vi "SetLimitTripOffLCDC501.vi"(2 "LASER LIMIT & TRIP-OFF":T1, 8 "error in (no error)":errorcluster, 11 "VISA resource name":refnum<visa-resource-name>) -> (0 "error out":errorcluster, 3 "VISA resource name out":refnum<visa-resource-name>)   [LabVIEW 2021]
panel:
  # "Laser Trip-off on"
  # "Current Limit"
  # "TEC Off"
  # "Min Temperature"
  # "Max Temperature"
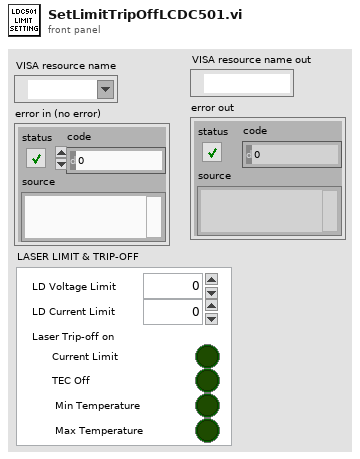
[diagram p1: front panel]
types:
  T1 = cluster{"LD Voltage Limit":dbl, "LD Current Limit":dbl, "Laser Trip-off on Current Limit":bool, "Laser Trip-off on TEC Off":bool, "Laser Trip-off on Min Temperature":bool, "Laser Trip-off on Max Temperature":bool}
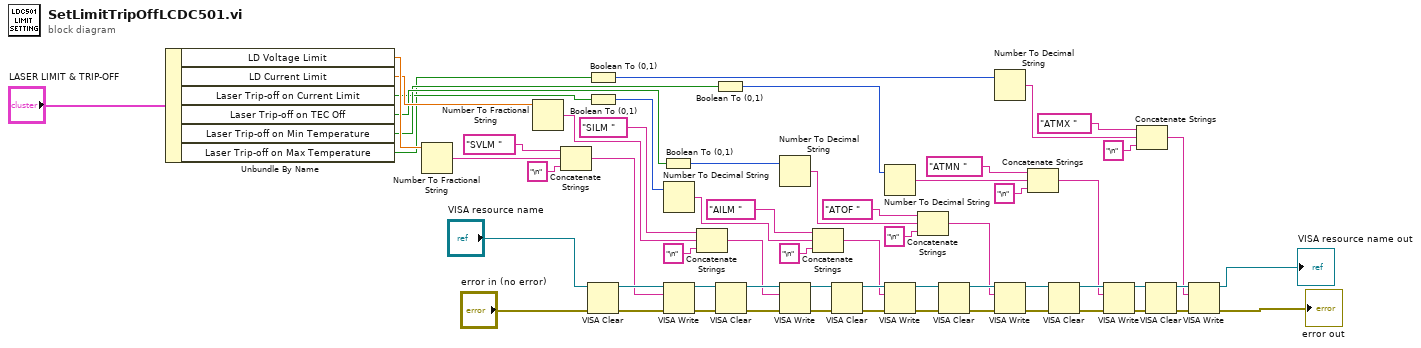
[diagram p0: block diagram]
diagram:
  n1 = Unbundle By Name("LASER LIMIT & TRIP-OFF") -> ("LD Voltage Limit"=w46:dbl, "LD Current Limit"=w45:dbl, "Laser Trip-off on Current Limit"=w42:bool, "Laser Trip-off on TEC Off"=w44:bool, "Laser Trip-off on Min Temperature"=w43:bool, "Laser Trip-off on Max Temperature"=w41:bool)
  n2 = Number To Fractional String(number=w46) -> (F-format string=w36:string)  [unwired: 3 in]
  n3 = Number To Fractional String(number=w45) -> (F-format string=w31:string)  [unwired: 3 in]
  n4 = Concatenate Strings("SVLM " ("write buffer"), w36, "\n" ("string")) -> (w33:string)
  n5 = Boolean To (0,1)(Boolean=w41) -> (0, 1=w37:i16)
  n6 = Boolean To (0,1)(Boolean=w42) -> (0, 1=w40:i16)
  n7 = VISA Clear(VISA resource name="VISA resource name", error in (no error)="error in (no error)") -> (VISA resource name out=w60:refnum<visa-resource-name>, error out=w61:errorcluster)
  n8 = Boolean To (0,1)(Boolean=w44) -> (0, 1=w39:i16)
  n9 = Number To Decimal String(number=w40) -> (decimal integer string=w22:string)  [unwired: 1 in]
  n10 = VISA Write(VISA resource name=w60, write buffer=w33, error in (no error)=w61) -> (VISA resource name out=w29:refnum<visa-resource-name>, error out=w28:errorcluster)  [unwired: 1 out]
  n11 = Concatenate Strings("SILM " ("write buffer"), w31, "\n" ("string")) -> (w27:string)
  n12 = Boolean To (0,1)(Boolean=w43) -> (0, 1=w38:i16)
  n13 = VISA Clear(VISA resource name=w29, error in (no error)=w28) -> (VISA resource name out=w58:refnum<visa-resource-name>, error out=w59:errorcluster)
  n14 = Number To Decimal String(number=w39) -> (decimal integer string=w17:string)  [unwired: 1 in]
  n15 = VISA Write(VISA resource name=w58, write buffer=w27, error in (no error)=w59) -> (VISA resource name out=w26:refnum<visa-resource-name>, error out=w25:errorcluster)  [unwired: 1 out]
  n16 = Concatenate Strings("AILM " ("write buffer"), w22, "\n" ("string")) -> (w21:string)
  n17 = VISA Clear(VISA resource name=w26, error in (no error)=w25) -> (VISA resource name out=w56:refnum<visa-resource-name>, error out=w57:errorcluster)
  n18 = Number To Decimal String(number=w38) -> (decimal integer string=w10:string)  [unwired: 1 in]
  n19 = VISA Write(VISA resource name=w56, write buffer=w21, error in (no error)=w57) -> (VISA resource name out=w20:refnum<visa-resource-name>, error out=w19:errorcluster)  [unwired: 1 out]
  n20 = Concatenate Strings("ATOF " ("write buffer"), w17, "\n" ("string")) -> (w15:string)
  n21 = VISA Clear(VISA resource name=w20, error in (no error)=w19) -> (VISA resource name out=w54:refnum<visa-resource-name>, error out=w55:errorcluster)
  n22 = Number To Decimal String(number=w37) -> (decimal integer string=w5:string)  [unwired: 1 in]
  n23 = VISA Write(VISA resource name=w54, write buffer=w15, error in (no error)=w55) -> (VISA resource name out=w13:refnum<visa-resource-name>, error out=w12:errorcluster)  [unwired: 1 out]
  n24 = Concatenate Strings("ATMN " ("write buffer"), w10, "\n" ("string")) -> (w9:string)
  n25 = VISA Clear(VISA resource name=w13, error in (no error)=w12) -> (VISA resource name out=w52:refnum<visa-resource-name>, error out=w53:errorcluster)
  n26 = VISA Write(VISA resource name=w52, write buffer=w9, error in (no error)=w53) -> (VISA resource name out=w7:refnum<visa-resource-name>, error out=w6:errorcluster)  [unwired: 1 out]
  n27 = Concatenate Strings("ATMX " ("string"), w5, "\n" ("string")) -> (w3:string)
  n28 = VISA Clear(VISA resource name=w7, error in (no error)=w6) -> (VISA resource name out=w50:refnum<visa-resource-name>, error out=w51:errorcluster)
  n29 = VISA Write(VISA resource name=w50, write buffer=w3, error in (no error)=w51) -> (VISA resource name out=→"VISA resource name out":refnum<visa-resource-name>, error out=→"error out":errorcluster)  [unwired: 1 out]
